vi "Calculate Manhattan Coverage.vi"(2 "Destination":T2, 3 "Origin":T2) -> (0 "Manhattan Distance":dbl, 1 "Coverage Area":T1)   [LabVIEW 2020, in "AoC 2022.lvlib"]
uses:
  AoC 2022.lvlib
  Location.ctl
  Coverage Area.ctl
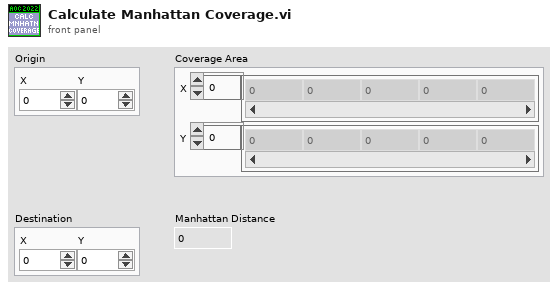
[diagram p1: front panel]
types:
  T1 = typedef "AoC 2022.lvlib/Coverage Area.ctl" = cluster{"X":dbl[], "Y":dbl[]}
  T2 = typedef "AoC 2022.lvlib/Location.ctl" = cluster{"X":i32, "Y":i32}
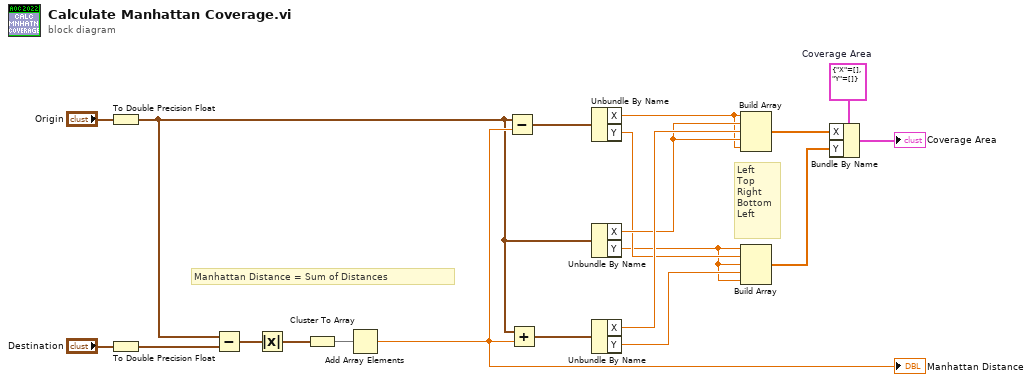
[diagram p0: block diagram]
diagram:
  w15 = T1 {"X"=[], "Y"=[]}  # Coverage Area
  # "Left\nTop\nRight\nBottom\nLeft"
  # "Manhattan Distance = Sum of Distances"
  n1 = To Double Precision Float(number="Origin") -> (double precision float=w9:cluster{"X":dbl, "Y":dbl})
  n2 = To Double Precision Float(number="Destination") -> (double precision float=w10:cluster{"X":dbl, "Y":dbl})
  n3 = Subtract(x=w9, y=w10) -> (x-y=w20:cluster{"X":dbl, "Y":dbl})
  n4 = Absolute Value(x=w20) -> (abs(x)=w19:cluster{"X":dbl, "Y":dbl})
  n5 = Cluster To Array(cluster=w19) -> (array=w18:dbl[])
  n6 = Add Array Elements(numeric array=w18) -> (sum=w17:dbl)
  "Manhattan Distance" <- w17
  n7 = Subtract(x=w9, y=w17) -> (x-y=w12:cluster{"X":dbl, "Y":dbl})
  n8 = Add(x=w9, y=w17) -> (x+y=w11:cluster{"X":dbl, "Y":dbl})
  n9 = Unbundle By Name(w12) -> ("X"=w2:dbl, "Y"=w3:dbl)
  n10 = Unbundle By Name(w9) -> ("X"=w5:dbl, "Y"=w1:dbl)
  n11 = Unbundle By Name(w11) -> ("X"=w6:dbl, "Y"=w4:dbl)
  n12 = Build Array(w2, w5, w6, w5, w2) -> (w8:dbl[])
  n13 = Build Array(w1, w3, w1, w4, w1) -> (w7:dbl[])
  n14 = Bundle By Name(cluster=w15, "X"=w8, "Y"=w7) -> (→"Coverage Area":T1)
